vi "PID2ChanGlobals.vi"() -> ()   [LabVIEW 2016]
panel:
  in  "Measured Pressures":dbl[](array[numeric])
  in  "Measured F0":dbl
  in  "Measured F1":dbl
  in  "Control On":bool
  in  "Use Control":bool
  in  "Measured Ratio":dbl
  in  "Set Ratio":dbl
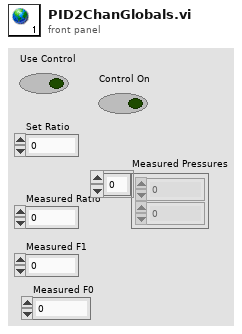
[diagram p1: front panel]
diagram:
